vi "VIP_Phase 1.vi"() -> ()   [LabVIEW 2024]
uses:
  <vilib>/DAQmx/read.llb/DAQmx Read (Digital 1D Bool 1Chan 1Samp).vi
  <vilib>/DAQmx/create/channels.llb/DAQmx Create Channel (DI-Digital Input).vi
  <vilib>/DAQmx/miscellaneous.llb/DAQmx Fill In Error Info.vi
  <vilib>/Utility/file.llb/Write To Spreadsheet File (DBL).vi
panel:
  out "Mouse file 4R":string
  out "Mouse file 3R":string
  out "Mouse file 2R":string
  out "Mouse file 1R":string
  out "mouse 4 R":cluster{"Y":dbl[], "Y":dbl[]}[](graph)
  out "mouse 4 L":cluster{"Y":dbl[], "Y":dbl[]}[](graph)
  out "mouse 3 R":cluster{"Y":dbl[], "Y":dbl[]}[](graph)
  out "mouse 3 L":cluster{"Y":dbl[], "Y":dbl[]}[](graph)
  out "mouse 2 R":cluster{"Y":dbl[], "Y":dbl[]}[](graph)
  out "mouse 2 L":cluster{"Y":dbl[], "Y":dbl[]}[](graph)
  in  "stop":bool
  out "4R":bool
  in  "fake 4R":bool
  out "water # 4R":dbl
  out "lick # 4R":dbl
  out "last water 4R":dbl
  out "state 4R":enum16{"waiting", "ITI"}(ring)
  in  "water port 4 R":tag="Dev1/port2/line0"
  in  "water dur (ms) 4R":dbl=11.0
  out "state 4L":enum16{"waiting", "ITI"}(ring)
  in  "fake 4L":bool
  out "4L":bool
  out "water # 4L":dbl
  out "lick # 4L":dbl
  out "last water 4L":dbl
  in  "water port 4 L":tag="Dev1/port1/line7"
  in  "water dur (ms) 4L":dbl=8.0
  in  "fake 3R":bool
  out "3R":bool
  out "state 3R":enum16{"waiting", "ITI"}(ring)
  out "water # 3R":dbl
  out "lick # 3R":dbl
  out "last water 3R":dbl
  in  "water port 3 R":tag="Dev1/port1/line6"
  in  "water dur (ms) 3R":dbl=28.0
  in  "fake 3L":bool
  out "3L":bool
  out "state 3L":enum16{"waiting", "ITI"}(ring)
  out "water # 3L":dbl
  out "lick # 3L":dbl
  out "last water 3L":dbl
  in  "water port 3 L":tag="Dev1/port1/line5"
  in  "water dur (ms) 3L":dbl=30.0
  in  "fake 2R":bool
  in  "fake 2L":bool
  in  "fake 1R":bool
  in  "fake 1L":bool
  out "mouse 1 R":cluster{"Y":dbl[], "Y":dbl[]}[](graph)
  out "mouse 1 L":cluster{"Y":dbl[], "Y":dbl[]}[](graph)
  out "2R":bool
  in  "Mouse ID 4":string="Test _4"
  out "Mouse file 4L":string
  out "state 2R":enum16{"waiting", "ITI"}(ring)
  out "water # 2R":dbl
  out "lick # 2R":dbl
  out "last water 2R":dbl
  in  "water port 2 R":tag="Dev1/port1/line4"
  in  "water dur (ms) 2R":dbl=24.5
  out "2L":bool
  in  "Mouse ID 3":string="Test_3"
  out "Mouse file 3L":string
  out "state 2L":enum16{"waiting", "ITI"}(ring)
  out "water # 2L":dbl
  out "lick # 2L":dbl
  out "last water 2L":dbl
  in  "water port 2 L":tag="Dev1/port1/line3"
  in  "water dur (ms) 2L":dbl=32.5
  out "1R":bool
  in  "Mouse ID 2":string="Test _2"
  out "last water 1R":dbl
  out "state 1R":enum16{"waiting", "ITI"}(ring)
  out "lick # 1R":dbl
  out "water # 1R":dbl
  out "Mouse file 2L":string
  in  "water port 1 R":tag="Dev1/port1/line2"
  in  "water dur (ms) 1R":dbl=23.0
  out "ITI (s)":dbl=9.0
  out "last water 1L":dbl
  out "1L":bool
  out "state 1L":enum16{"waiting", "ITI"}(ring)
  out "water # 1L":dbl
  out "lick # 1L":dbl
  in  "water dur (ms) 1L":dbl=30.0
  in  "water port1 L":tag="Dev1/port1/line1"
  out "Mouse file 1L":string
  out "data folder":path=path "C:/Users/congy/Desktop/Gritton Lab/LabVIEW_Practical/LabVIEW Data"
  in  "Mouse ID 1":string="Test_1"
  out "time (s)":dbl
  in  "lick port":tag="Dev1/port0/line0:7"
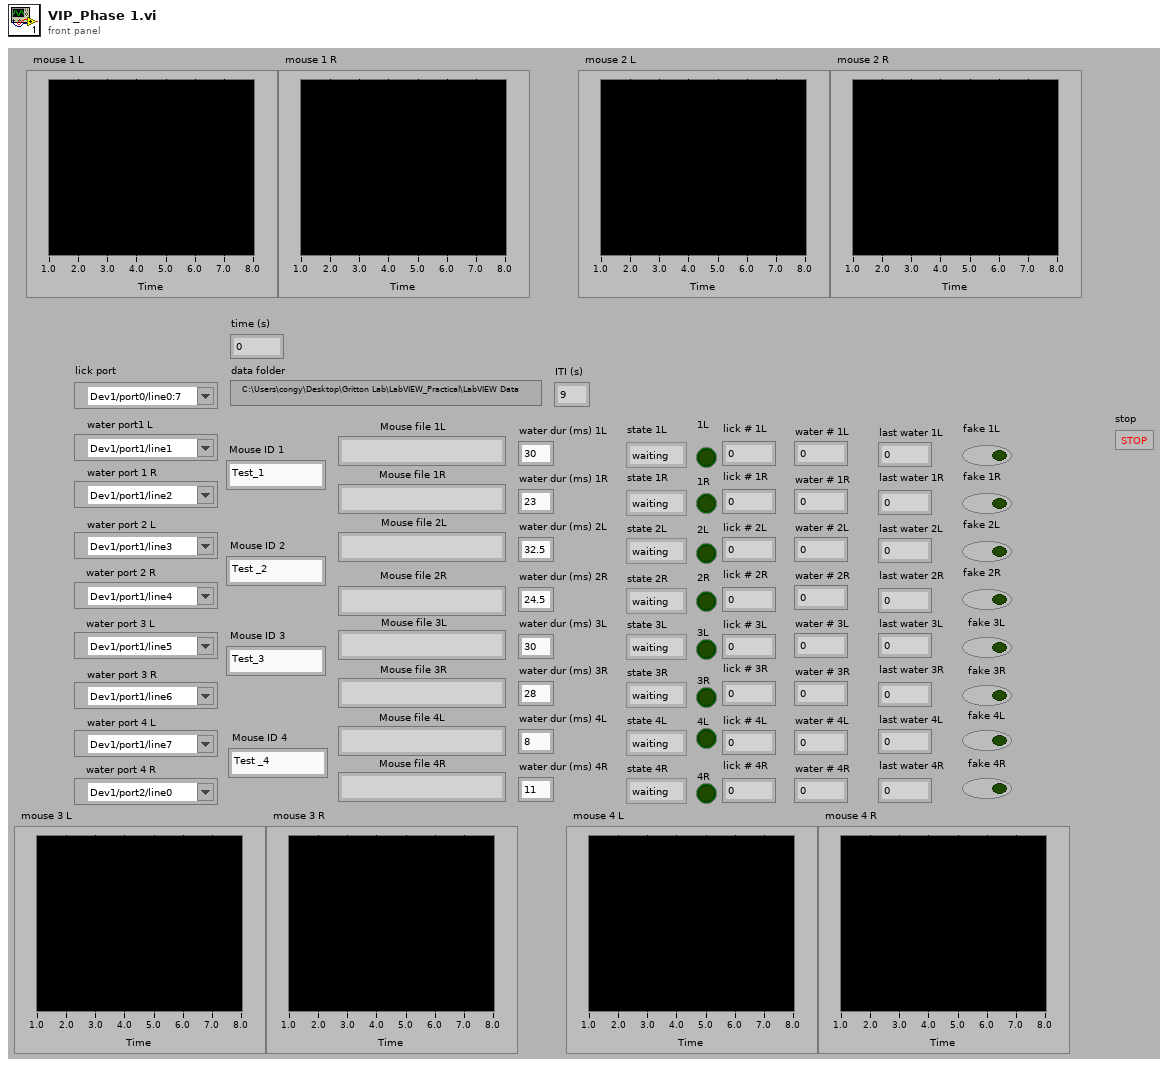
[diagram p1: front panel]
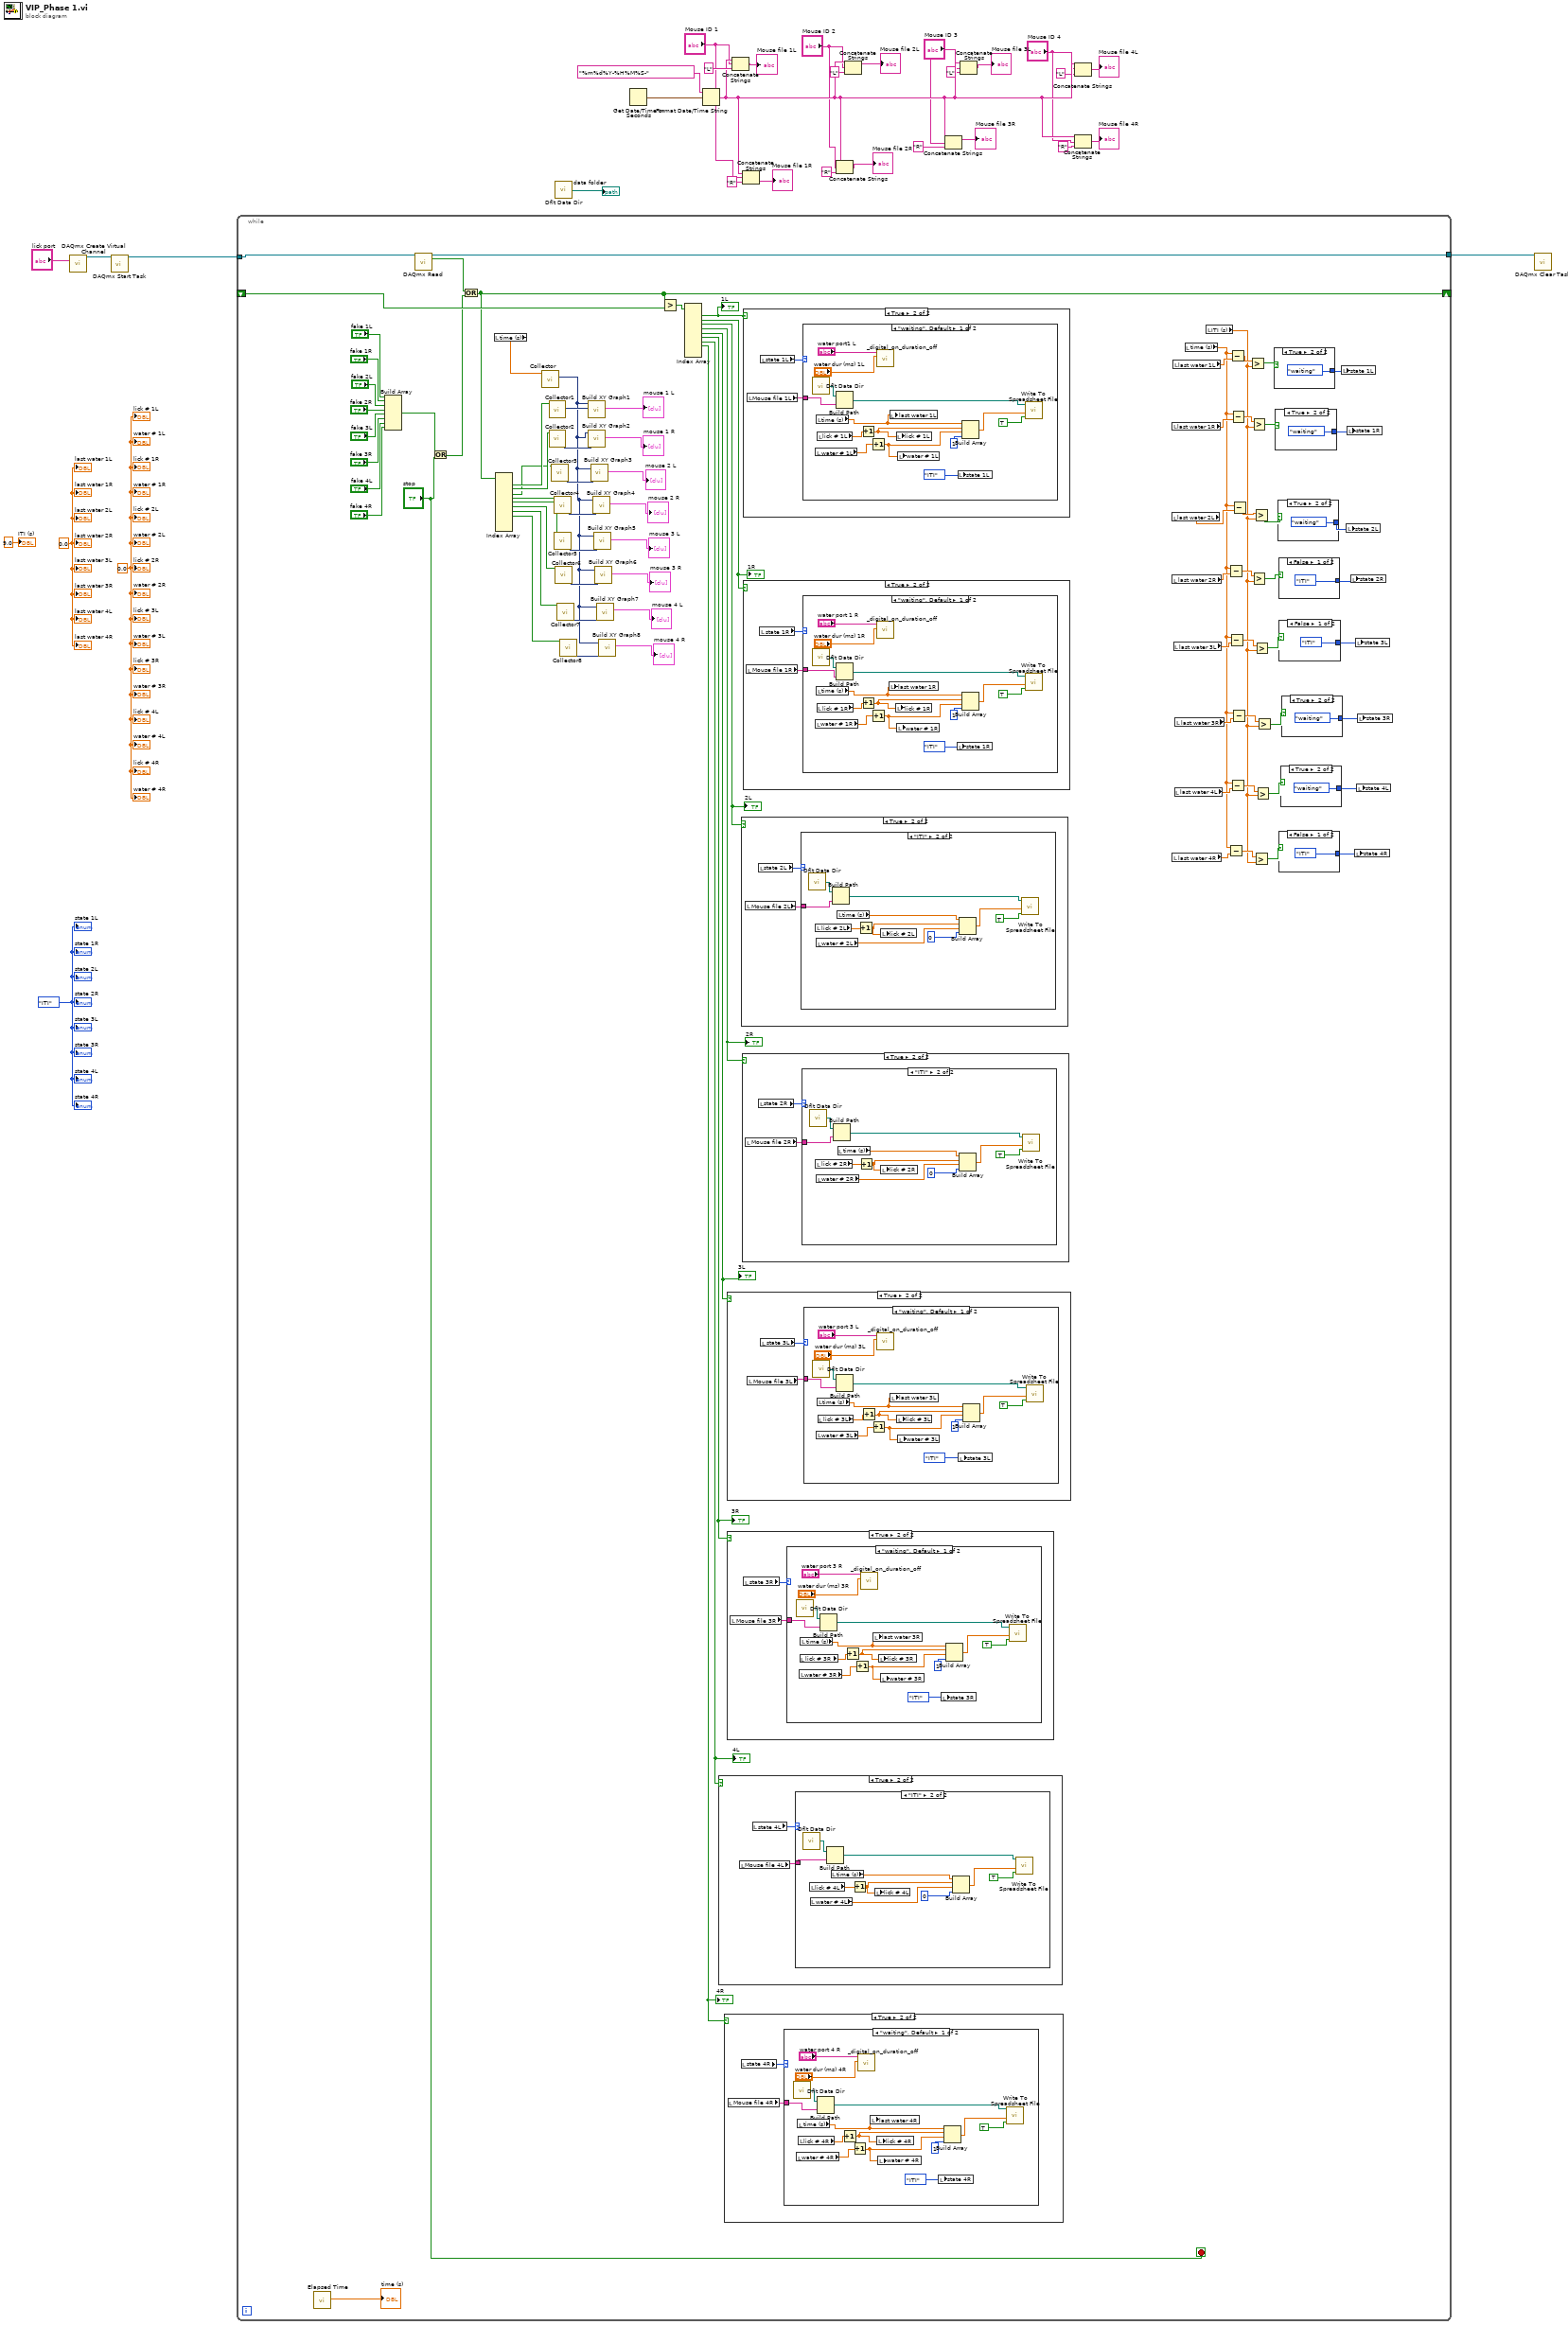
[diagram p0: block diagram]
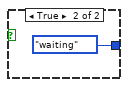
[diagram p2: hidden frame]
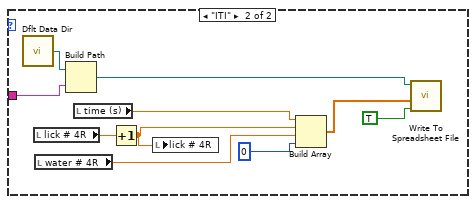
[diagram p4: hidden frame]
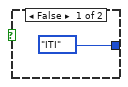
[diagram p5: hidden frame]
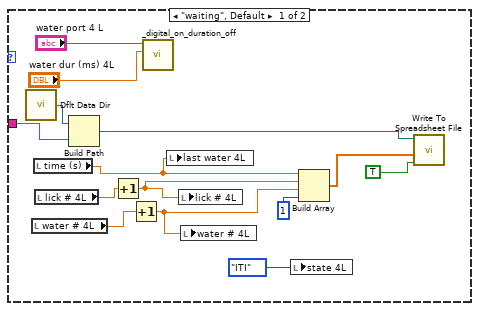
[diagram p7: hidden frame]
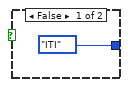
[diagram p8: hidden frame]
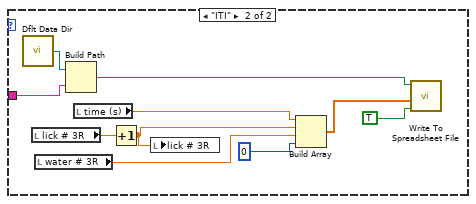
[diagram p10: hidden frame]
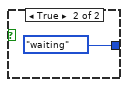
[diagram p11: hidden frame]
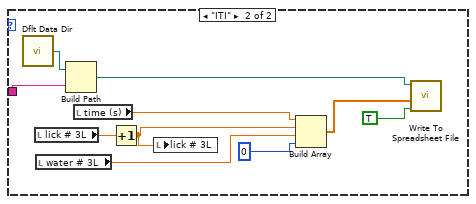
[diagram p13: hidden frame]
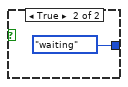
[diagram p14: hidden frame]
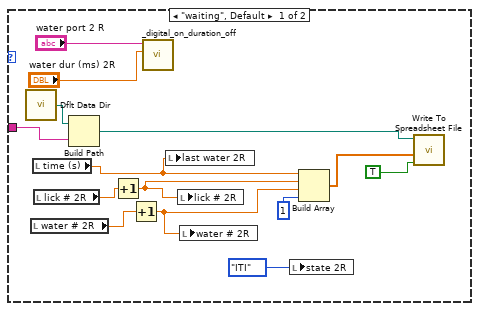
[diagram p16: hidden frame]
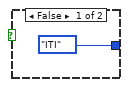
[diagram p17: hidden frame]
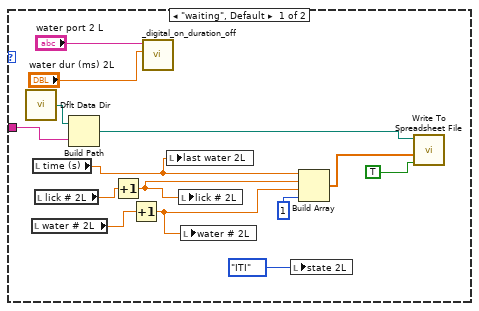
[diagram p19: hidden frame]
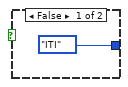
[diagram p20: hidden frame]
diagram:
  w20 = 0.0 ("last water 1L")
  w19 = 0.0
  w18 = enum16{"waiting", "ITI"}."ITI"
  n1 = call-poly <vilib>:"DAQmx Create Virtual Channel.vi"("lines"="lick port") -> ("task out"=w31:refnum<k21>)  [unwired: 13 in, 1 out]
  n2 = call <vilib>:"DAQmx Start Task.vi"("task/channels in"=w31) -> ("task out"=w30:refnum<k21>)  [unwired: 13 in, 1 out]
  n3 = while {
    tunnel: w30 -> [w118]
    tunnel: [w117] -> w29
    shift-right: [w81] -> _
    shift-left: _ -> [w116]
    stop <- "stop" stop-if-true
    n4 = call "Elapsed Time"() -> ("Elapsed Time (s)"=→"time (s)":dbl)  [unwired: 12 in, 7 out]
    n5 = Build Array("fake 1L", "fake 1R", "fake 2L", "fake 2R", "fake 3L", "fake 3R", "fake 4L", "fake 4R") -> (w54:bool[])
    n6 = call-poly <vilib>:"DAQmx Read.vi"("task/channels in"=w118) -> ("task out"=w117:refnum<k21>, "data"=w82:bool[])  [unwired: 12 in, 1 out]
    n7 = Or(x=w54, y="stop") -> (x .or. y?=w53:bool[])
    n8 = Or(x=w82, y=w53) -> (x .or. y?=w81:bool[])
    n9 = local read "time (s)"() -> (w96:dbl)
    n10 = Index Array(array=w81) -> (element #1=w95:bool, element #2=w93:bool, element #3=w49:bool, element #4=w46:bool, element #5=w43:bool, element #6=w40:bool, element #7=w37:bool, element #8=w33:bool)  [unwired: 11 in, 3 out]
    n11 = call "Collector"("Signals"=w96) -> ("Collected Signals"=w34:dynamicdata)  [unwired: 9 in, 1 out]
    n12 = call "Collector1"("Signals"=w95) -> ("Collected Signals"=w97:dynamicdata)  [unwired: 9 in, 1 out]
    n13 = call "Collector2"("Signals"=w93) -> ("Collected Signals"=w94:dynamicdata)  [unwired: 9 in, 1 out]
    n14 = call "Collector3"("Signals"=w49) -> ("Collected Signals"=w51:dynamicdata)  [unwired: 9 in, 1 out]
    n15 = call "Collector4"("Signals"=w46) -> ("Collected Signals"=w48:dynamicdata)  [unwired: 9 in, 1 out]
    n16 = call "Collector5"("Signals"=w43) -> ("Collected Signals"=w45:dynamicdata)  [unwired: 9 in, 1 out]
    n17 = call "Collector6"("Signals"=w40) -> ("Collected Signals"=w42:dynamicdata)  [unwired: 9 in, 1 out]
    n18 = call "Collector7"("Signals"=w37) -> ("Collected Signals"=w39:dynamicdata)  [unwired: 9 in, 1 out]
    n19 = call "Collector8"("Signals"=w33) -> ("Collected Signals"=w36:dynamicdata)  [unwired: 9 in, 1 out]
    n20 = call "Build XY Graph1"("Y Input"=w97, "X Input"=w34) -> ("XY Graph"=→"mouse 1 L":cluster{"Y":dbl[], "Y":dbl[]}[])  [unwired: 3 in, 6 out]
    n21 = call "Build XY Graph2"("Y Input"=w94, "X Input"=w34) -> ("XY Graph"=→"mouse 1 R":cluster{"Y":dbl[], "Y":dbl[]}[])  [unwired: 3 in, 6 out]
    n22 = call "Build XY Graph3"("Y Input"=w51, "X Input"=w34) -> ("XY Graph"=→"mouse 2 L":cluster{"Y":dbl[], "Y":dbl[]}[])  [unwired: 3 in, 6 out]
    n23 = call "Build XY Graph4"("Y Input"=w48, "X Input"=w34) -> ("XY Graph"=→"mouse 2 R":cluster{"Y":dbl[], "Y":dbl[]}[])  [unwired: 3 in, 6 out]
    n24 = call "Build XY Graph5"("Y Input"=w45, "X Input"=w34) -> ("XY Graph"=→"mouse 3 L":cluster{"Y":dbl[], "Y":dbl[]}[])  [unwired: 3 in, 6 out]
    n25 = call "Build XY Graph6"("Y Input"=w42, "X Input"=w34) -> ("XY Graph"=→"mouse 3 R":cluster{"Y":dbl[], "Y":dbl[]}[])  [unwired: 3 in, 6 out]
    n26 = call "Build XY Graph7"("Y Input"=w39, "X Input"=w34) -> ("XY Graph"=→"mouse 4 L":cluster{"Y":dbl[], "Y":dbl[]}[])  [unwired: 3 in, 6 out]
    n27 = call "Build XY Graph8"("Y Input"=w36, "X Input"=w34) -> ("XY Graph"=→"mouse 4 R":cluster{"Y":dbl[], "Y":dbl[]}[])  [unwired: 3 in, 6 out]
    n28 = Greater?(x=w81, y=w116) -> (0:w114:bool[])
    n29 = Index Array(array=w114) -> (element #1=w113:bool, element #2=w104:bool, element #3=w99:bool, element #4=w98:bool, element #5=w80:bool, element #6=w74:bool, element #7=w68:bool, element #8=w61:bool)  [unwired: 10 in, 2 out]
    "1L" <- w113
    "1R" <- w104
    "2L" <- w99
    "2R" <- w98
    "3L" <- w80
    "3R" <- w74
    "4L" <- w68
    "4R" <- w61
    n30 = case shown="True" w68 {
      frame False {
      }
      frame True {
        n31 = local read "Mouse file 4L"() -> (w149:string)
        n32 = local read "state 4L"() -> (w150:enum16{"waiting", "ITI"})
        n33 = case shown="\"ITI\"" w150 {
          tunnel: w149 -> [w160 w165]
          frame "waiting", Default {
            n34 = call <vilib>:"Dflt Data Dir.vi"() -> ("App:Default Data Directory"=w161:path)
            n35 = local read "water # 4L"() -> (w157:dbl)
            n36 = local read "time (s)"() -> (w151:dbl)
            n37 = local read "lick # 4L"() -> (w158:dbl)
            n38 = Build Path(base path=w161, name or relative path=w160) -> (appended path=w159:path)
            n39 = Increment(x=w158) -> (x+1=w153:dbl)
            n40 = Increment(x=w157) -> (x+1=w152:dbl)
            n41 = call "_digital_on_duration_off.vi"("duration (ms)"="water dur (ms) 4L", "digital port"="water port 4 L") -> ()  [unwired: 10 in]
            n42 = local write "last water 4L"(w151) -> ()
            n43 = local write "lick # 4L"(w153) -> ()
            n44 = local write "water # 4L"(w152) -> ()
            n45 = local write "state 4L"(enum16{"waiting", "ITI"}."ITI") -> ()
            n46 = Build Array(w151, w153, w152, 1) -> (w155:dbl[])
            n47 = call-poly <vilib>:"Write To Spreadsheet File.vi"("append to file? (new file:F)"=TRUE, "1D data"=w155, "file path (dialog if empty)"=w159) -> ()  [unwired: 5 in, 1 out]
          }
          frame "ITI" {
            n48 = call <vilib>:"Dflt Data Dir.vi"() -> ("App:Default Data Directory"=w174:path)
            n49 = local read "lick # 4L"() -> (w167:dbl)
            n50 = local read "water # 4L"() -> (w169:dbl)
            n51 = Build Path(base path=w174, name or relative path=w165) -> (appended path=w172:path)
            n52 = local read "time (s)"() -> (w170:dbl)
            n53 = Increment(x=w167) -> (x+1=w166:dbl)
            n54 = local write "lick # 4L"(w166) -> ()
            n55 = Build Array(w170, w166, w169, 0) -> (w171:dbl[])
            n56 = call-poly <vilib>:"Write To Spreadsheet File.vi"("append to file? (new file:F)"=TRUE, "1D data"=w171, "file path (dialog if empty)"=w172) -> ()  [unwired: 5 in, 1 out]
          }
        }
      }
    }
    n57 = case shown="True" w61 {
      frame False {
      }
      frame True {
        n58 = local read "Mouse file 4R"() -> (w121:string)
        n59 = local read "state 4R"() -> (w122:enum16{"waiting", "ITI"})
        n60 = case shown="\"waiting\", Default" w122 {
          tunnel: w121 -> [w132 w145]
          frame "waiting", Default {
            n61 = call <vilib>:"Dflt Data Dir.vi"() -> ("App:Default Data Directory"=w133:path)
            n62 = local read "water # 4R"() -> (w129:dbl)
            n63 = local read "time (s)"() -> (w123:dbl)
            n64 = local read "lick # 4R"() -> (w130:dbl)
            n65 = Build Path(base path=w133, name or relative path=w132) -> (appended path=w131:path)
            n66 = Increment(x=w130) -> (x+1=w125:dbl)
            n67 = Increment(x=w129) -> (x+1=w124:dbl)
            n68 = call "_digital_on_duration_off.vi"("duration (ms)"="water dur (ms) 4R", "digital port"="water port 4 R") -> ()  [unwired: 10 in]
            n69 = local write "last water 4R"(w123) -> ()
            n70 = local write "lick # 4R"(w125) -> ()
            n71 = local write "water # 4R"(w124) -> ()
            n72 = local write "state 4R"(enum16{"waiting", "ITI"}."ITI") -> ()
            n73 = Build Array(w123, w125, w124, 1) -> (w127:dbl[])
            n74 = call-poly <vilib>:"Write To Spreadsheet File.vi"("append to file? (new file:F)"=TRUE, "1D data"=w127, "file path (dialog if empty)"=w131) -> ()  [unwired: 5 in, 1 out]
          }
          frame "ITI" {
            n75 = call <vilib>:"Dflt Data Dir.vi"() -> ("App:Default Data Directory"=w146:path)
            n76 = local read "lick # 4R"() -> (w138:dbl)
            n77 = local read "water # 4R"() -> (w140:dbl)
            n78 = Build Path(base path=w146, name or relative path=w145) -> (appended path=w143:path)
            n79 = local read "time (s)"() -> (w141:dbl)
            n80 = Increment(x=w138) -> (x+1=w137:dbl)
            n81 = local write "lick # 4R"(w137) -> ()
            n82 = Build Array(w141, w137, w140, 0) -> (w142:dbl[])
            n83 = call-poly <vilib>:"Write To Spreadsheet File.vi"("append to file? (new file:F)"=TRUE, "1D data"=w142, "file path (dialog if empty)"=w143) -> ()  [unwired: 5 in, 1 out]
          }
        }
      }
    }
    n84 = case shown="True" w80 {
      frame False {
      }
      frame True {
        n85 = local read "Mouse file 3L"() -> (w205:string)
        n86 = local read "state 3L"() -> (w206:enum16{"waiting", "ITI"})
        n87 = case shown="\"waiting\", Default" w206 {
          tunnel: w205 -> [w216 w221]
          frame "waiting", Default {
            n88 = call <vilib>:"Dflt Data Dir.vi"() -> ("App:Default Data Directory"=w217:path)
            n89 = local read "water # 3L"() -> (w213:dbl)
            n90 = local read "time (s)"() -> (w207:dbl)
            n91 = local read "lick # 3L"() -> (w214:dbl)
            n92 = Build Path(base path=w217, name or relative path=w216) -> (appended path=w215:path)
            n93 = Increment(x=w214) -> (x+1=w209:dbl)
            n94 = Increment(x=w213) -> (x+1=w208:dbl)
            n95 = call "_digital_on_duration_off.vi"("duration (ms)"="water dur (ms) 3L", "digital port"="water port 3 L") -> ()  [unwired: 10 in]
            n96 = local write "last water 3L"(w207) -> ()
            n97 = local write "lick # 3L"(w209) -> ()
            n98 = local write "water # 3L"(w208) -> ()
            n99 = local write "state 3L"(enum16{"waiting", "ITI"}."ITI") -> ()
            n100 = Build Array(w207, w209, w208, 1) -> (w211:dbl[])
            n101 = call-poly <vilib>:"Write To Spreadsheet File.vi"("append to file? (new file:F)"=TRUE, "1D data"=w211, "file path (dialog if empty)"=w215) -> ()  [unwired: 5 in, 1 out]
          }
          frame "ITI" {
            n102 = call <vilib>:"Dflt Data Dir.vi"() -> ("App:Default Data Directory"=w230:path)
            n103 = local read "lick # 3L"() -> (w223:dbl)
            n104 = local read "water # 3L"() -> (w225:dbl)
            n105 = Build Path(base path=w230, name or relative path=w221) -> (appended path=w228:path)
            n106 = local read "time (s)"() -> (w226:dbl)
            n107 = Increment(x=w223) -> (x+1=w222:dbl)
            n108 = local write "lick # 3L"(w222) -> ()
            n109 = Build Array(w226, w222, w225, 0) -> (w227:dbl[])
            n110 = call-poly <vilib>:"Write To Spreadsheet File.vi"("append to file? (new file:F)"=TRUE, "1D data"=w227, "file path (dialog if empty)"=w228) -> ()  [unwired: 5 in, 1 out]
          }
        }
      }
    }
    n111 = case shown="True" w74 {
      frame False {
      }
      frame True {
        n112 = local read "Mouse file 3R"() -> (w177:string)
        n113 = local read "state 3R"() -> (w178:enum16{"waiting", "ITI"})
        n114 = case shown="\"waiting\", Default" w178 {
          tunnel: w177 -> [w188 w201]
          frame "waiting", Default {
            n115 = call <vilib>:"Dflt Data Dir.vi"() -> ("App:Default Data Directory"=w189:path)
            n116 = local read "water # 3R"() -> (w185:dbl)
            n117 = local read "lick # 3R"() -> (w186:dbl)
            n118 = local read "time (s)"() -> (w179:dbl)
            n119 = Build Path(base path=w189, name or relative path=w188) -> (appended path=w187:path)
            n120 = Increment(x=w186) -> (x+1=w181:dbl)
            n121 = Increment(x=w185) -> (x+1=w180:dbl)
            n122 = call "_digital_on_duration_off.vi"("duration (ms)"="water dur (ms) 3R", "digital port"="water port 3 R") -> ()  [unwired: 10 in]
            n123 = local write "last water 3R"(w179) -> ()
            n124 = local write "lick # 3R"(w181) -> ()
            n125 = local write "water # 3R"(w180) -> ()
            n126 = local write "state 3R"(enum16{"waiting", "ITI"}."ITI") -> ()
            n127 = Build Array(w179, w181, w180, 1) -> (w183:dbl[])
            n128 = call-poly <vilib>:"Write To Spreadsheet File.vi"("append to file? (new file:F)"=TRUE, "1D data"=w183, "file path (dialog if empty)"=w187) -> ()  [unwired: 5 in, 1 out]
          }
          frame "ITI" {
            n129 = call <vilib>:"Dflt Data Dir.vi"() -> ("App:Default Data Directory"=w202:path)
            n130 = local read "lick # 3R"() -> (w194:dbl)
            n131 = local read "water # 3R"() -> (w196:dbl)
            n132 = Build Path(base path=w202, name or relative path=w201) -> (appended path=w199:path)
            n133 = local read "time (s)"() -> (w197:dbl)
            n134 = Increment(x=w194) -> (x+1=w193:dbl)
            n135 = local write "lick # 3R"(w193) -> ()
            n136 = Build Array(w197, w193, w196, 0) -> (w198:dbl[])
            n137 = call-poly <vilib>:"Write To Spreadsheet File.vi"("append to file? (new file:F)"=TRUE, "1D data"=w198, "file path (dialog if empty)"=w199) -> ()  [unwired: 5 in, 1 out]
          }
        }
      }
    }
    n138 = case shown="True" w99 {
      frame False {
      }
      frame True {
        n139 = local read "Mouse file 2L"() -> (w261:string)
        n140 = local read "state 2L"() -> (w262:enum16{"waiting", "ITI"})
        n141 = case shown="\"ITI\"" w262 {
          tunnel: w261 -> [w272 w285]
          frame "waiting", Default {
            n142 = call <vilib>:"Dflt Data Dir.vi"() -> ("App:Default Data Directory"=w273:path)
            n143 = local read "water # 2L"() -> (w269:dbl)
            n144 = local read "time (s)"() -> (w263:dbl)
            n145 = local read "lick # 2L"() -> (w270:dbl)
            n146 = Build Path(base path=w273, name or relative path=w272) -> (appended path=w271:path)
            n147 = Increment(x=w270) -> (x+1=w265:dbl)
            n148 = Increment(x=w269) -> (x+1=w264:dbl)
            n149 = call "_digital_on_duration_off.vi"("duration (ms)"="water dur (ms) 2L", "digital port"="water port 2 L") -> ()  [unwired: 10 in]
            n150 = local write "last water 2L"(w263) -> ()
            n151 = local write "lick # 2L"(w265) -> ()
            n152 = local write "water # 2L"(w264) -> ()
            n153 = local write "state 2L"(enum16{"waiting", "ITI"}."ITI") -> ()
            n154 = Build Array(w263, w265, w264, 1) -> (w267:dbl[])
            n155 = call-poly <vilib>:"Write To Spreadsheet File.vi"("append to file? (new file:F)"=TRUE, "1D data"=w267, "file path (dialog if empty)"=w271) -> ()  [unwired: 5 in, 1 out]
          }
          frame "ITI" {
            n156 = call <vilib>:"Dflt Data Dir.vi"() -> ("App:Default Data Directory"=w286:path)
            n157 = local read "lick # 2L"() -> (w278:dbl)
            n158 = local read "water # 2L"() -> (w280:dbl)
            n159 = Build Path(base path=w286, name or relative path=w285) -> (appended path=w283:path)
            n160 = local read "time (s)"() -> (w281:dbl)
            n161 = Increment(x=w278) -> (x+1=w277:dbl)
            n162 = local write "lick # 2L"(w277) -> ()
            n163 = Build Array(w281, w277, w280, 0) -> (w282:dbl[])
            n164 = call-poly <vilib>:"Write To Spreadsheet File.vi"("append to file? (new file:F)"=TRUE, "1D data"=w282, "file path (dialog if empty)"=w283) -> ()  [unwired: 5 in, 1 out]
          }
        }
      }
    }
    n165 = case shown="True" w98 {
      frame False {
      }
      frame True {
        n166 = local read "Mouse file 2R"() -> (w233:string)
        n167 = local read "state 2R"() -> (w234:enum16{"waiting", "ITI"})
        n168 = case shown="\"ITI\"" w234 {
          tunnel: w233 -> [w244 w257]
          frame "waiting", Default {
            n169 = call <vilib>:"Dflt Data Dir.vi"() -> ("App:Default Data Directory"=w245:path)
            n170 = local read "water # 2R"() -> (w241:dbl)
            n171 = local read "time (s)"() -> (w235:dbl)
            n172 = local read "lick # 2R"() -> (w242:dbl)
            n173 = Build Path(base path=w245, name or relative path=w244) -> (appended path=w243:path)
            n174 = Increment(x=w242) -> (x+1=w237:dbl)
            n175 = Increment(x=w241) -> (x+1=w236:dbl)
            n176 = call "_digital_on_duration_off.vi"("duration (ms)"="water dur (ms) 2R", "digital port"="water port 2 R") -> ()  [unwired: 10 in]
            n177 = local write "last water 2R"(w235) -> ()
            n178 = local write "lick # 2R"(w237) -> ()
            n179 = local write "water # 2R"(w236) -> ()
            n180 = local write "state 2R"(enum16{"waiting", "ITI"}."ITI") -> ()
            n181 = Build Array(w235, w237, w236, 1) -> (w239:dbl[])
            n182 = call-poly <vilib>:"Write To Spreadsheet File.vi"("append to file? (new file:F)"=TRUE, "1D data"=w239, "file path (dialog if empty)"=w243) -> ()  [unwired: 5 in, 1 out]
          }
          frame "ITI" {
            n183 = call <vilib>:"Dflt Data Dir.vi"() -> ("App:Default Data Directory"=w258:path)
            n184 = local read "lick # 2R"() -> (w250:dbl)
            n185 = local read "water # 2R"() -> (w252:dbl)
            n186 = Build Path(base path=w258, name or relative path=w257) -> (appended path=w255:path)
            n187 = local read "time (s)"() -> (w253:dbl)
            n188 = Increment(x=w250) -> (x+1=w249:dbl)
            n189 = local write "lick # 2R"(w249) -> ()
            n190 = Build Array(w253, w249, w252, 0) -> (w254:dbl[])
            n191 = call-poly <vilib>:"Write To Spreadsheet File.vi"("append to file? (new file:F)"=TRUE, "1D data"=w254, "file path (dialog if empty)"=w255) -> ()  [unwired: 5 in, 1 out]
          }
        }
      }
    }
    n192 = case shown="True" w113 {
      frame False {
      }
      frame True {
        n193 = local read "Mouse file 1L"() -> (w317:string)
        n194 = local read "state 1L"() -> (w318:enum16{"waiting", "ITI"})
        n195 = case shown="\"waiting\", Default" w318 {
          tunnel: w317 -> [w328 w341]
          frame "waiting", Default {
            n196 = call <vilib>:"Dflt Data Dir.vi"() -> ("App:Default Data Directory"=w329:path)
            n197 = local read "water # 1L"() -> (w325:dbl)
            n198 = local read "time (s)"() -> (w319:dbl)
            n199 = local read "lick # 1L"() -> (w326:dbl)
            n200 = Build Path(base path=w329, name or relative path=w328) -> (appended path=w327:path)
            n201 = Increment(x=w326) -> (x+1=w321:dbl)
            n202 = Increment(x=w325) -> (x+1=w320:dbl)
            n203 = call "_digital_on_duration_off.vi"("duration (ms)"="water dur (ms) 1L", "digital port"="water port1 L") -> ()  [unwired: 10 in]
            n204 = local write "last water 1L"(w319) -> ()
            n205 = local write "lick # 1L"(w321) -> ()
            n206 = local write "water # 1L"(w320) -> ()
            n207 = local write "state 1L"(enum16{"waiting", "ITI"}."ITI") -> ()
            n208 = Build Array(w319, w321, w320, 1) -> (w323:dbl[])
            n209 = call-poly <vilib>:"Write To Spreadsheet File.vi"("append to file? (new file:F)"=TRUE, "1D data"=w323, "file path (dialog if empty)"=w327) -> ()  [unwired: 5 in, 1 out]
          }
          frame "ITI" {
            n210 = call <vilib>:"Dflt Data Dir.vi"() -> ("App:Default Data Directory"=w342:path)
            n211 = local read "lick # 1L"() -> (w334:dbl)
            n212 = local read "water # 1L"() -> (w336:dbl)
            n213 = Build Path(base path=w342, name or relative path=w341) -> (appended path=w339:path)
            n214 = local read "time (s)"() -> (w337:dbl)
            n215 = Increment(x=w334) -> (x+1=w333:dbl)
            n216 = local write "lick # 1L"(w333) -> ()
            n217 = Build Array(w337, w333, w336, 0) -> (w338:dbl[])
            n218 = call-poly <vilib>:"Write To Spreadsheet File.vi"("append to file? (new file:F)"=TRUE, "1D data"=w338, "file path (dialog if empty)"=w339) -> ()  [unwired: 5 in, 1 out]
          }
        }
      }
    }
    n219 = case shown="True" w104 {
      frame False {
      }
      frame True {
        n220 = local read "Mouse file 1R"() -> (w289:string)
        n221 = local read "state 1R"() -> (w290:enum16{"waiting", "ITI"})
        n222 = case shown="\"waiting\", Default" w290 {
          tunnel: w289 -> [w291 w313]
          frame "waiting", Default {
            n223 = call <vilib>:"Dflt Data Dir.vi"() -> ("App:Default Data Directory"=w301:path)
            n224 = local read "water # 1R"() -> (w298:dbl)
            n225 = local read "time (s)"() -> (w292:dbl)
            n226 = local read "lick # 1R"() -> (w299:dbl)
            n227 = Build Path(base path=w301, name or relative path=w291) -> (appended path=w300:path)
            n228 = Increment(x=w299) -> (x+1=w294:dbl)
            n229 = Increment(x=w298) -> (x+1=w293:dbl)
            n230 = call "_digital_on_duration_off.vi"("duration (ms)"="water dur (ms) 1R", "digital port"="water port 1 R") -> ()  [unwired: 10 in]
            n231 = local write "last water 1R"(w292) -> ()
            n232 = local write "lick # 1R"(w294) -> ()
            n233 = local write "water # 1R"(w293) -> ()
            n234 = local write "state 1R"(enum16{"waiting", "ITI"}."ITI") -> ()
            n235 = Build Array(w292, w294, w293, 1) -> (w296:dbl[])
            n236 = call-poly <vilib>:"Write To Spreadsheet File.vi"("append to file? (new file:F)"=TRUE, "1D data"=w296, "file path (dialog if empty)"=w300) -> ()  [unwired: 5 in, 1 out]
          }
          frame "ITI" {
            n237 = call <vilib>:"Dflt Data Dir.vi"() -> ("App:Default Data Directory"=w314:path)
            n238 = local read "lick # 1R"() -> (w306:dbl)
            n239 = local read "water # 1R"() -> (w308:dbl)
            n240 = Build Path(base path=w314, name or relative path=w313) -> (appended path=w311:path)
            n241 = local read "time (s)"() -> (w309:dbl)
            n242 = Increment(x=w306) -> (x+1=w305:dbl)
            n243 = local write "lick # 1R"(w305) -> ()
            n244 = Build Array(w309, w305, w308, 0) -> (w310:dbl[])
            n245 = call-poly <vilib>:"Write To Spreadsheet File.vi"("append to file? (new file:F)"=TRUE, "1D data"=w310, "file path (dialog if empty)"=w311) -> ()  [unwired: 5 in, 1 out]
          }
        }
      }
    }
    n246 = local read "last water 1R"() -> (w106:dbl)
    n247 = local read "last water 2L"() -> (w101:dbl)
    n248 = local read "last water 2R"() -> (w88:dbl)
    n249 = local read "last water 4R"() -> (w59:dbl)
    n250 = local read "last water 1L"() -> (w111:dbl)
    n251 = local read "last water 3L"() -> (w78:dbl)
    n252 = local read "last water 4L"() -> (w65:dbl)
    n253 = local read "last water 3R"() -> (w71:dbl)
    n254 = local read "time (s)"() -> (w56:dbl)
    n255 = local read "ITI (s)"() -> (w55:dbl)
    n256 = Subtract(x=w56, y=w88) -> (x-y=w89:dbl)
    n257 = Subtract(x=w56, y=w59) -> (x-y=w58:dbl)
    n258 = Subtract(x=w56, y=w78) -> (x-y=w77:dbl)
    n259 = Subtract(x=w56, y=w111) -> (x-y=w110:dbl)
    n260 = Subtract(x=w56, y=w65) -> (x-y=w64:dbl)
    n261 = Subtract(x=w56, y=w106) -> (x-y=w107:dbl)
    n262 = Subtract(x=w56, y=w71) -> (x-y=w70:dbl)
    n263 = Subtract(x=w56, y=w101) -> (x-y=w102:dbl)
    n264 = Greater?(x=w110, y=w55) -> (0:w112:bool)
    n265 = Greater?(x=w107, y=w55) -> (0:w108:bool)
    n266 = Greater?(x=w89, y=w55) -> (0:w90:bool)
    n267 = Greater?(x=w102, y=w55) -> (0:w103:bool)
    n268 = Greater?(x=w58, y=w55) -> (0:w57:bool)
    n269 = Greater?(x=w77, y=w55) -> (0:w76:bool)
    n270 = Greater?(x=w64, y=w55) -> (0:w63:bool)
    n271 = Greater?(x=w70, y=w55) -> (0:w69:bool)
    n272 = case shown="True" w112 {
      tunnel: [enum16{"waiting", "water", "ITI"}."ITI" enum16{"waiting", "ITI"}."waiting"] -> w109
      frame False {
      }
      frame True {
      }
    }
    n273 = case shown="True" w108 {
      tunnel: [enum16{"waiting", "water", "ITI"}."ITI" enum16{"waiting", "ITI"}."waiting"] -> w105
      frame False {
      }
      frame True {
      }
    }
    n274 = case shown="True" w103 {
      tunnel: [enum16{"waiting", "water", "ITI"}."ITI" enum16{"waiting", "ITI"}."waiting"] -> w100
      frame False {
      }
      frame True {
      }
    }
    n275 = case shown="False" w90 {
      tunnel: [enum16{"waiting", "water", "ITI"}."ITI" enum16{"waiting", "ITI"}."waiting"] -> w87
      frame False {
      }
      frame True {
      }
    }
    n276 = case shown="False" w57 {
      tunnel: [enum16{"waiting", "water", "ITI"}."ITI" enum16{"waiting", "ITI"}."waiting"] -> w60
      frame False {
      }
      frame True {
      }
    }
    n277 = case shown="False" w76 {
      tunnel: [enum16{"waiting", "ITI"}."ITI" enum16{"waiting", "water", "ITI"}."waiting"] -> w79
      frame False {
      }
      frame True {
      }
    }
    n278 = case shown="True" w63 {
      tunnel: [enum16{"waiting", "water", "ITI"}."ITI" enum16{"waiting", "ITI"}."waiting"] -> w66
      frame False {
      }
      frame True {
      }
    }
    n279 = case shown="True" w69 {
      tunnel: [enum16{"waiting", "water", "ITI"}."ITI" enum16{"waiting", "ITI"}."waiting"] -> w72
      frame False {
      }
      frame True {
      }
    }
    n280 = local write "state 1L"(w109) -> ()
    n281 = local write "state 2L"(w100) -> ()
    n282 = local write "state 1R"(w105) -> ()
    n283 = local write "state 2R"(w87) -> ()
    n284 = local write "state 4R"(w60) -> ()
    n285 = local write "state 3L"(w79) -> ()
    n286 = local write "state 4L"(w66) -> ()
    n287 = local write "state 3R"(w72) -> ()
  }
  n288 = call <vilib>:"Dflt Data Dir.vi"() -> ("App:Default Data Directory"=→"data folder":path)
  n289 = Get Date/Time In Seconds() -> (seconds since 1Jan1904=w28:timestamp)
  n290 = Format Date/Time String(time format string (%c)="%m%d%Y-%H%M%S-", seconds (now)=w28) -> (date/time string=w9:string)  [unwired: 1 in]
  n291 = Concatenate Strings(w9, "Mouse ID 1", "L" ("string")) -> (→"Mouse file 1L":string)
  n292 = Concatenate Strings(w9, "Mouse ID 1", "R" ("string")) -> (→"Mouse file 1R":string)
  n293 = Concatenate Strings(w9, "Mouse ID 2", "R" ("string")) -> (→"Mouse file 2R":string)
  n294 = Concatenate Strings(w9, "Mouse ID 2", "L" ("string")) -> (→"Mouse file 2L":string)
  n295 = Concatenate Strings(w9, "Mouse ID 3", "R" ("string")) -> (→"Mouse file 3R":string)
  n296 = Concatenate Strings(w9, "Mouse ID 3", "L" ("string")) -> (→"Mouse file 3L":string)
  n297 = Concatenate Strings(w9, "Mouse ID 4", "L" ("string")) -> (→"Mouse file 4L":string)
  n298 = Concatenate Strings(w9, "Mouse ID 4", "R" ("string")) -> (→"Mouse file 4R":string)
  n299 = call <vilib>:"DAQmx Clear Task.vi"("task in"=w29) -> ()  [unwired: 14 in, 1 out]
  "water # 1L" <- w19
  "lick # 1L" <- w19
  "state 1L" <- w18
  "last water 1L" <- w20
  "ITI (s)" <- 9.0 ("ITI (s)")
  "last water 1R" <- w20
  "lick # 1R" <- w19
  "water # 1R" <- w19
  "state 1R" <- w18
  "last water 2L" <- w20
  "lick # 2L" <- w19
  "water # 2L" <- w19
  "state 2L" <- w18
  "last water 2R" <- w20
  "lick # 2R" <- w19
  "water # 2R" <- w19
  "state 2R" <- w18
  "state 3L" <- w18
  "last water 3L" <- w20
  "lick # 3L" <- w19
  "water # 3L" <- w19
  "state 3R" <- w18
  "last water 3R" <- w20
  "lick # 3R" <- w19
  "water # 3R" <- w19
  "last water 4L" <- w20
  "lick # 4L" <- w19
  "water # 4L" <- w19
  "state 4L" <- w18
  "state 4R" <- w18
  "last water 4R" <- w20
  "lick # 4R" <- w19
  "water # 4R" <- w19
